vi "Begin.vi"(8 "error in":errorcluster) -> (0 "error out":errorcluster)   [LabVIEW 2019]
doc: "Called before other user functions, this VI is expected to open initial I/O refnums, load in file data, and do all program initialization. Notice that the <B>error out</B> terminal is simply used for data flow. Wiring it to other structures or subVIs ensures that this VI runs first."
uses:
  <vilib>/Rock Robotics/WPI/Solenoid/WPI_SolenoidOpenSingle.vi
  <vilib>/Rock Robotics/WPI/Joystick/WPI_JoystickDeviceEnum.ctl
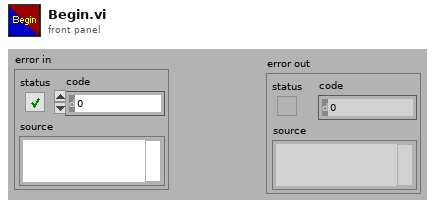
[diagram p1: front panel]
types:
  T1 = typedef "WPI_JoystickDeviceEnum.ctl" = enum16{"USB 0", "USB 1", "USB 2", "USB 3", "USB 4", "USB 5"}
  T2 = typedef "WPI_SolenoidDevRef.ctl" = cluster{"DevStatus":errorcluster, "Pneumatics Control Module":u8, "Forward Solenoid Channel":T3, "Reverse Solenoid Channel":T3}
  T3 = typedef "WPI_SolenoidChannel.ctl" = enum8{"Solenoid 0", "Solenoid 1", "Solenoid 2", "Solenoid 3", "Solenoid 4", "Solenoid 5", "Solenoid 6", "Solenoid 7", "Invalid"}
  T4 = typedef "WPI_CompressorDevRef.ctl" = cluster{"DevStatus":errorcluster, "Pneumatics Control Module":u8}
  T5 = typedef "WPI_JoystickDevRef.ctl" = cluster{"Device":T1}
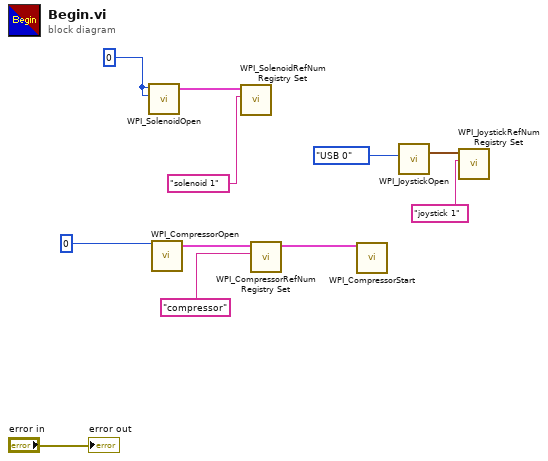
[diagram p0: block diagram]
diagram:
  w5 = 0
  n1 = call-poly <vilib>:"WPI_SolenoidOpen.vi"("Solenoid Channel"=w5, "Pneumatics Control Module (0)"=w5) -> ("SolenoidDevRef"=w6:T2)  [unwired: 8 in, 1 out]
  n2 = call <vilib>:"WPI_CompressorOpen.vi"("Pneumatics Control Module (0)"=0) -> ("CompressorDevRef"=w9:T4)  [unwired: 13 in, 1 out]
  n3 = call <vilib>:"WPI_SolenoidRefNum Registry Set.vi"("refnum name"="solenoid 1", "SolenoidDevRef"=w6) -> ()  [unwired: 8 in, 2 out]
  n4 = call <vilib>:"WPI_CompressorRefNum Registry Set.vi"("refnum name"="compressor", "CompressorDevRef"=w9) -> ("CompressorDevRef"=w7:T4)  [unwired: 8 in, 1 out]
  n5 = call <vilib>:"WPI_CompressorStart.vi"("CompressorDevRef"=w7) -> ()  [unwired: 9 in, 2 out]
  n6 = call <vilib>:"WPI_JoystickOpen.vi"("JoystickDevice"=WPI_JoystickDeviceEnum."USB 0") -> ("JoystickDevRef"=w3:T5)  [unwired: 10 in]
  n7 = call <vilib>:"WPI_JoystickRefNum Registry Set.vi"("refnum name"="joystick 1", "JoystickDevRef"=w3) -> ()  [unwired: 8 in, 2 out]
  "error out" <- "error in"
